vi "RT-ANN-Node.vi"(1 "Weights OutputSize x (InputSize + 1)":dbl[][](array[numeric]), 2 "Input":dbl[](array[numeric]), 3 "Size of Output":i32) -> (0 "Output":dbl[](array[numeric]))   [LabVIEW 2020]
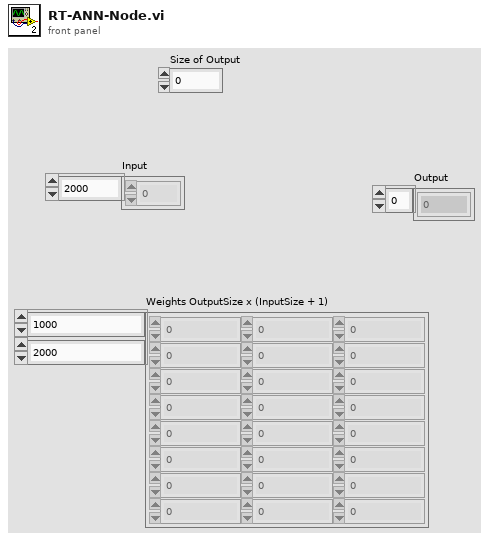
[diagram p1: front panel]
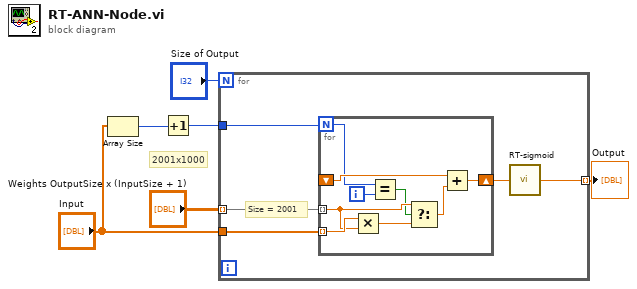
[diagram p0: block diagram]
diagram:
  # "2001x1000"
  n1 = Array Size(array="Input") -> (size(s)=w2:i32)
  n2 = Increment(x=w2) -> (x+1=w1:i32)
  n3 = for {
    N: "Size of Output" -> [_]
    tunnel: w1 -> [w11]
    tunnel: "Input" -> [w10]
    tunnel: "Weights OutputSize x (InputSize + 1)" -> [w9] mode=indexing
    tunnel: [w7] -> w3 mode=indexing
    # "Size = 2001"
    n4 = for {
      N: w11 -> [w13]
      shift-right: [w19] -> w8
      shift-left: _ -> [w20]
      tunnel: w10 -> [w18] mode=indexing
      tunnel: w9 -> [w17] mode=indexing
      i -> [w14]
      n5 = Multiply(x=w18, y=w17) -> (x*y=w16:dbl)
      n6 = Equal?(x=w13, y=w14) -> (x = y?=w12:bool)
      n7 = Select(t=w17, s=w12, f=w16) -> (s? t:f=w15:dbl)
      n8 = Add(x=w20, y=w15) -> (x+y=w19:dbl)
    }
    n9 = call "RT-sigmoid.vi"("x"=w8) -> ("Sigmoid"=w7:dbl)
  }
  "Output" <- w3
